vi "fgvExp.vi"(8 "error in":errorcluster, 11 "Enum":enum16{"set", "read", "close"}(ring)) -> (0 "error out":errorcluster, 3 "Image Out fgv":T1(plugin-control))   [LabVIEW 2018]
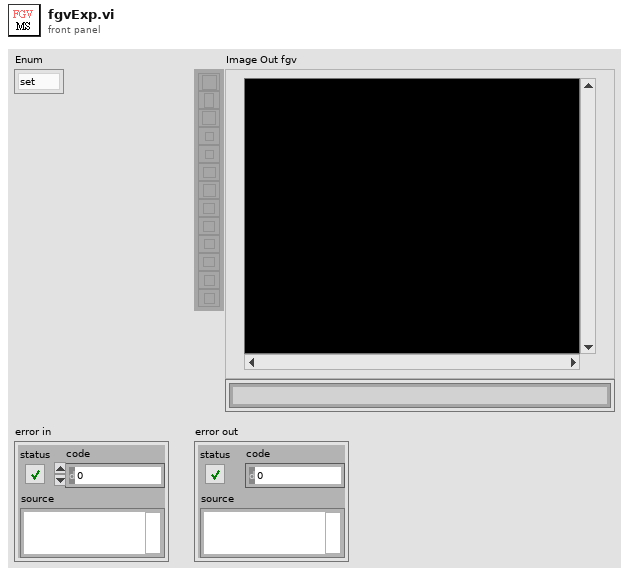
[diagram p1: front panel]
types:
  T1 = typedef "IMAQ Image.ctl" = refnum<image>
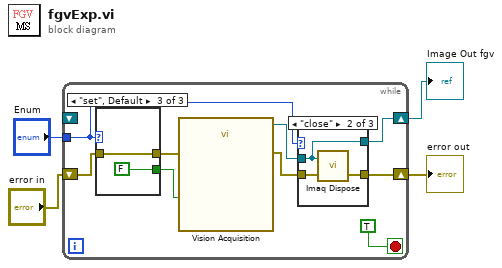
[diagram p0: block diagram]
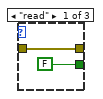
[diagram p4: hidden frame]
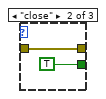
[diagram p5: hidden frame]
diagram:
  n1 = while {
    tunnel: "Enum" -> [w5]
    shift-right: [w11] -> w3
    shift-left: "error in" -> [w10]
    shift-right: [w6] -> w1
    shift-left: _ -> [_]
    stop <- TRUE stop-if-true
    n2 = case shown="\"set\", Default" w5 {
      tunnel: [w21 w24 w25] -> w9
      tunnel: [FALSE ("Stop (F)") TRUE ("Stop (F)") FALSE ("Stop (F)")] -> w12
      tunnel: w10 -> [w21 w24 w25]
      frame "read" {
      }
      frame "close" {
      }
      frame "set", Default {
      }
    }
    n3 = call "Vision Acquisition"("Stop (F)"=w12, "error in"=w9) -> ("Image Out"=w7:T1, "error out"=w8:errorcluster)  [unwired: 23 in, 1 out]
    n4 = case shown="\"close\"" w5 {
      tunnel: [w15 w18 w19] -> w11
      tunnel: w8 -> [w15 w17 w19]
      tunnel: w7 -> [w14 w16 w20]
      tunnel: [w14 w16 w20] -> w6
      frame "read" {
      }
      frame "close" {
        n5 = call "Imaq Dispose"("Image"=w16, "error in (no error)"=w17) -> ("error out"=w18:errorcluster)  [unwired: 4 in]
      }
      frame Default {
      }
    }
  }
  "Image Out fgv" <- w1
  "error out" <- w3
